vi "Logger.FindData.vi"() -> ()   [LabVIEW 2016]
uses:
  Global/ApplicationGlobal.vi
panel:
  in  "Folder":path
  out "size(s) 2":i32
  in  "Time from":timestamp=timestamp(3573842400 s since 1904-01-01)
  out "size(s)":i32
  out "error in (no error) 2":errorcluster
  out "Files":path[](array[path])
  in  "error in (no error)":errorcluster
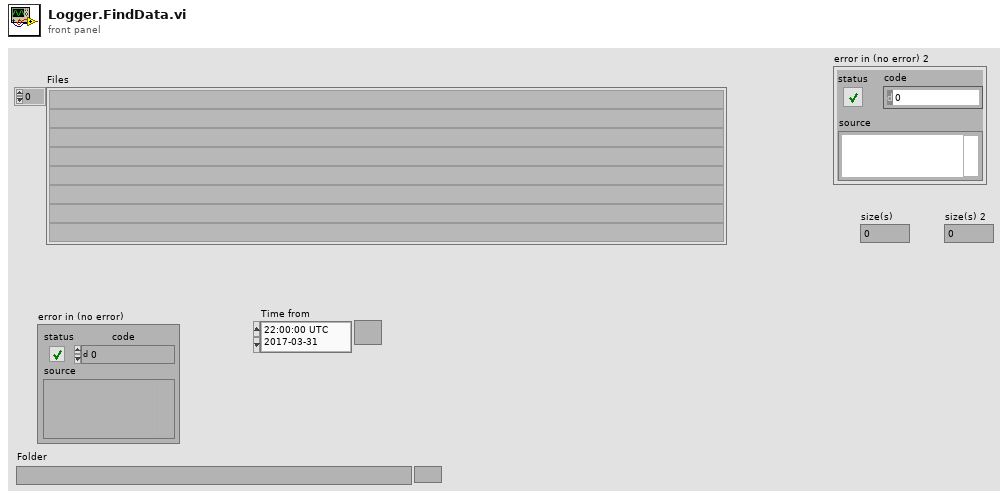
[diagram p1: front panel]
types:
  T1 = typedef "Logger.File.ctl" = cluster{"Props":T2, "Data":T5[]}
  T2 = typedef "Logger.File.Properties.ctl" = cluster{"FilePath":path, "ImgFolder":string, "Ref":string, "Serial":string, "SerialFormat":T3, "Duration":dbl, "Time From":timestamp, "Time To":timestamp, "Service":bool, "IgnoreImgs":bool, "CheckDMC":bool, "Counters":T4, "Err":errorcluster}
  T3 = typedef "Sequence.Code.SerialFormat.ctl" = enum8{"", "6 dig", "7 dig"}
  T4 = typedef "Sequence.Counters.ctl" = cluster{"Expected":u16, "Done":u16, "OK":u16, "NOK":u16, "NOKlimit":u16, "Part":u16, "PartOK":u16}
  T5 = typedef "Logger.File.Serials.ctl" = cluster{"TS from":timestamp, "TS to":timestamp, "SlotID":u8, "StatusA":T6, "SerialA":string, "CodeA":string, "ImgA":string, "CornersA":cluster{"X":i32, "Y":i32}[], "verificationA":u8, "StatusB":T6, "SerialB":string, "CodeB":string, "ImgB":string, "CornersB":cluster{"X":i32, "Y":i32}[], "verificationB":u8}
  T6 = typedef "Sequence.Step.Status.ctl" = enum16{"-", "Pending", "Running", "Skipped", "Passed", "Failed", "Done", "Error", "Aborted", "Stopped"}
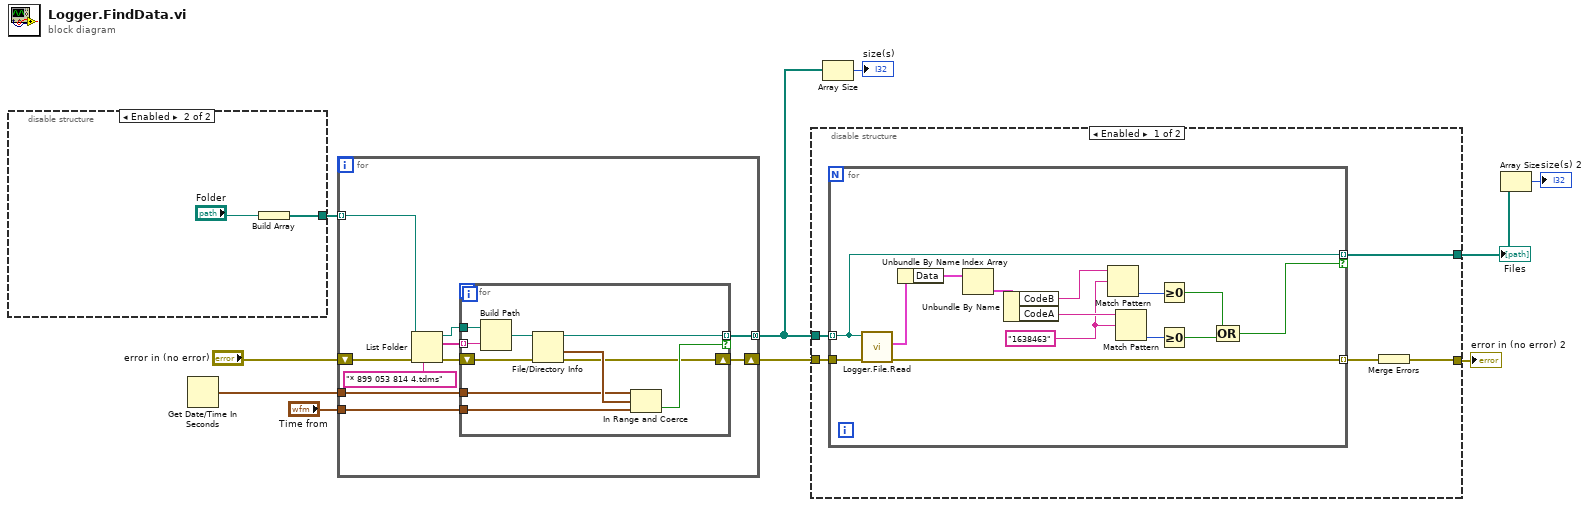
[diagram p0: block diagram]
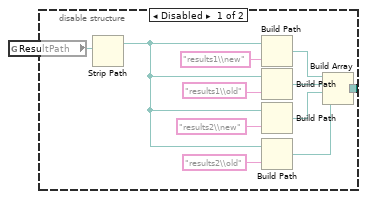
[diagram p2: hidden frame]
diagram:
  n1 = disable-structure shown="Enabled" {
    disable-tunnel: [w20 w22] -> w10
    frame Disabled {
      n2 = global read "ApplicationGlobal.vi" "ResultPath"() -> (w18:path)
      n3 = Strip Path(path=w18) -> (stripped path=w13:path)  [unwired: 1 out]
      n4 = Build Path(base path=w13, name or relative path="results1\\new") -> (appended path=w21:path)
      n5 = Build Path(base path=w13, name or relative path="results1\\old") -> (appended path=w19:path)
      n6 = Build Path(base path=w13, name or relative path="results2\\new") -> (appended path=w12:path)
      n7 = Build Path(base path=w13, name or relative path="results2\\old") -> (appended path=w11:path)
      n8 = Build Array(w21, w19, w12, w11) -> (w20:path[])
    }
    frame Enabled {
      n9 = Build Array("Folder") -> (w22:path[])
    }
  }
  n10 = Get Date/Time In Seconds() -> (seconds since 1Jan1904=w3:timestamp)
  n11 = for {
    tunnel: w10 -> [w32] mode=indexing
    tunnel: [w28] -> w6 mode=concatenating
    shift-right: [w26] -> w8
    shift-left: "error in (no error)" -> [w33]
    tunnel: "Time from" -> [w25]
    tunnel: w3 -> [w24]
    n12 = List Folder(path=w32, pattern="* 899 053 814 4.tdms", error in=w33) -> (path out=w30:path, filenames=w31:string[], error out=w27:errorcluster)  [unwired: 1 in, 1 out]
    n13 = for {
      tunnel: w31 -> [w43] mode=indexing
      tunnel: w30 -> [w42]
      tunnel: [w39] -> w28 mode=indexing if=w35
      shift-right: [w34] -> w26
      shift-left: w27 -> [w41]
      tunnel: w25 -> [w37]
      tunnel: w24 -> [w36]
      n14 = Build Path(base path=w42, name or relative path=w43) -> (appended path=w40:path)
      n15 = File/Directory Info(path=w40, error in=w41) -> (path out=w39:path, last mod=w38:timestamp, error out=w34:errorcluster)  [unwired: 4 out]
      n16 = In Range and Coerce(upper limit=w36, x=w38, lower limit=w37) -> (In Range?=w35:bool)  [unwired: 1 out]
    }
  }
  n17 = disable-structure shown="Enabled" {
    disable-tunnel: w8 -> [w48 w63]
    disable-tunnel: w6 -> [w47 _]
    disable-tunnel: [w44 w63] -> w7
    disable-tunnel: [w46 _] -> w1
    frame Enabled {
      n18 = for {
        tunnel: w48 -> [w62]
        tunnel: w47 -> [w59] mode=indexing
        tunnel: [w59] -> w46 mode=indexing if=w50
        tunnel: [w55] -> w45 mode=indexing
        w52 = "1638463" ("regular expression")
        n19 = call "Logger.File.Read.vi"("error in (no error)"=w62, "file path"=w59) -> ("error out"=w55:errorcluster, "File content"=w54:T1)  [unwired: 6 in, 2 out]
        n20 = Unbundle By Name(w54) -> ("Data"=w61:T5[])
        n21 = Index Array(array=w61) -> (element=w60:T5)  [unwired: 1 in]
        n22 = Unbundle By Name(w60) -> ("CodeB"=w53:string, "CodeA"=w58:string)
        n23 = Match Pattern(string=w53, regular expression=w52) -> (offset past match=w51:i32)  [unwired: 1 in, 3 out]
        n24 = Match Pattern(string=w58, regular expression=w52) -> (offset past match=w57:i32)  [unwired: 1 in, 3 out]
        n25 = Greater Or Equal To 0?(x=w51) -> (x >= 0?=w49:bool)
        n26 = Greater Or Equal To 0?(x=w57) -> (x >= 0?=w56:bool)
        n27 = Compound Arithmetic op=OR(w49, w56) -> (w50:bool)
      }
      n28 = Merge Errors(w45) -> (w44:errorcluster)
    }
    frame Disabled {
    }
  }
  "error in (no error) 2" <- w7
  "Files" <- w1
  n29 = Array Size(array=w6) -> (size(s)=→"size(s)":i32)
  n30 = Array Size(array=w1) -> (size(s)=→"size(s) 2":i32)
